vi "Get My Own Process ID.vi"(4 "Error In":errorcluster) -> (0 "Error Out":errorcluster, 3 "PID":u16)   [LabVIEW 2014, in "Managing Executables.lvlib"]
uses:
  Managing Executables.lvlib
  kernel32.dll
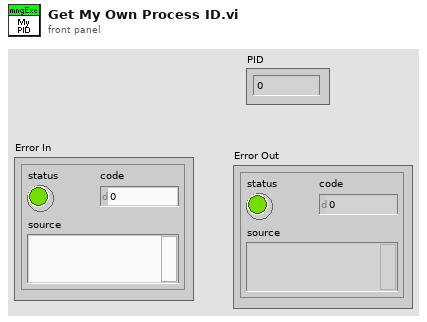
[diagram p1: front panel]
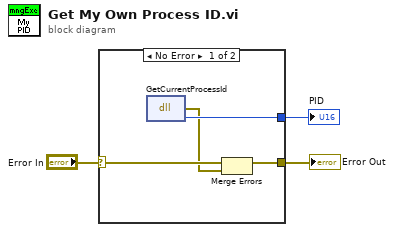
[diagram p0: block diagram]
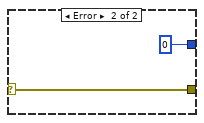
[diagram p2: hidden frame]
diagram:
  n1 = case shown="No Error" "Error In" {
    selector: "Error In" -> [w6 w9]
    tunnel: [w7 u16 0 ("return type")] -> w3
    tunnel: [w5 w9] -> w1
    frame No Error {
      n2 = dll-call lib="kernel32.dll" fn="GetCurrentProcessId"() -> (error out=w4:errorcluster, "return type"=w7:u16)  [unwired: 3 in, 1 out]
      n3 = Merge Errors(w6, w4) -> (w5:errorcluster)
    }
    frame Error {
    }
  }
  "PID" <- w3
  "Error Out" <- w1
